vi "DtCreateCtrFreqChan.vi"(5 "Board Name":string, 7 "Counter Num":u32, 9 "Input Line":i32(ring) items=["ClockInput", "GateInput"], 11 "error in (no error)":errorcluster) -> (4 "Task out":i32, 15 "error out":errorcluster)   [LabVIEW 2016]
doc: "Creates one or more virtual counter/timer channels that measure the frequency, in kHz, of an external digital signal that is connected to the counter/timer's clock input or gate input source.\n\nNote that internally, this VI measures the frequency of the input line based on two consecutive rising edges on the specified input line. Therefore, to use this VI your device must support edge-to-edge measurement mode.\n\nOnce you have created a virtual counter/timer channel for a frequency measurement task, you can start the task and read the frequency using the DtOLRead (Read Single Channel - Single Sample) VI."
uses:
  <userlib>/LV-Link3/DtLvLink.lvlib
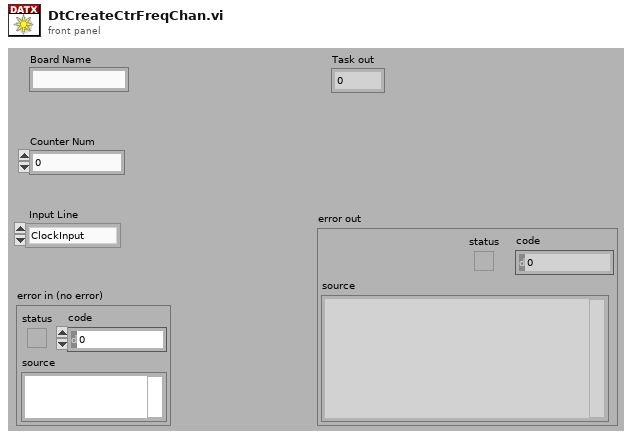
[diagram p1: front panel]
types:
  T1 = enum32{"AnalogInput", "AnalogOutput", "DigitalInput", "DigitalOutput", "Quadrature", "CounterTimer"}
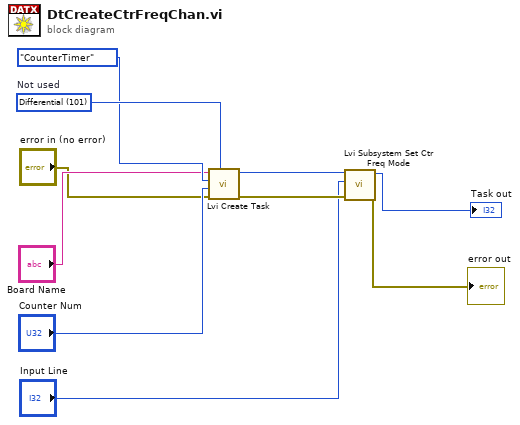
[diagram p0: block diagram]
diagram:
  w10 = 101 items=["SingleEnded"=100, "Differential"=101]  # Not used
  n1 = call <userlib>:"Lvi Create Task.vi"("SEorDiff"=w10, "error in (no error)"="error in (no error)", "SubSysIndex"="Counter Num", "ChanType"=T1."CounterTimer", "BoardName"="Board Name") -> ("error out"=w2:errorcluster, "TaskRef"=w5:i32)  [unwired: 4 in, 1 out]
  n2 = call <userlib>:"Lvi Subsystem Set Ctr Freq Mode.vi"("error in (no error)"=w2, "InputLine"="Input Line", "TaskRef"=w5) -> ("error out"=→"error out":errorcluster, "TaskRef out"=→"Task out":i32)  [unwired: 6 in, 1 out]
